vi "Template - Queue1.vi"(7 "Queue Selector":T2=enum."EnQ", 8 "error in (no error)":errorcluster, 10 "Queue1 Data":cluster{"Enum":T1, "Variant":variant}) -> (0 "error out":errorcluster, 2 "Queue Data (out)":cluster{"Enum":T1, "Variant":variant}, 3 "Q1 Ref":T3)   [LabVIEW 2012]
uses:
  TypeDef - Template - Q1 Ref.ctl
  TypeDef - Template - Queue1 Data Enum.ctl
  Navistar Library/Controls/TypeDef - Queue Selector(Standard).ctl
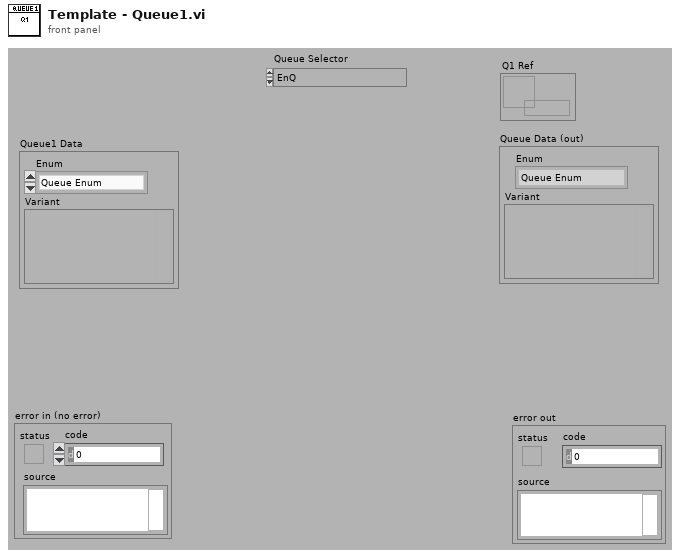
[diagram p1: front panel]
types:
  T1 = typedef "TypeDef - Template - Queue1 Data Enum.ctl" = enum16{"Queue Enum", "Get Time Data", "Check Time", "Stop"}
  T2 = typedef "TypeDef - Queue Selector(Standard).ctl" = enum16{"Create Q", "EnQ", "EnQ at the Opposite", "Flush Q", "Get Q Ref", "Clear Q", "Reset Q"}
  T3 = typedef "TypeDef - Template - Q1 Ref.ctl" = refnum<queue>
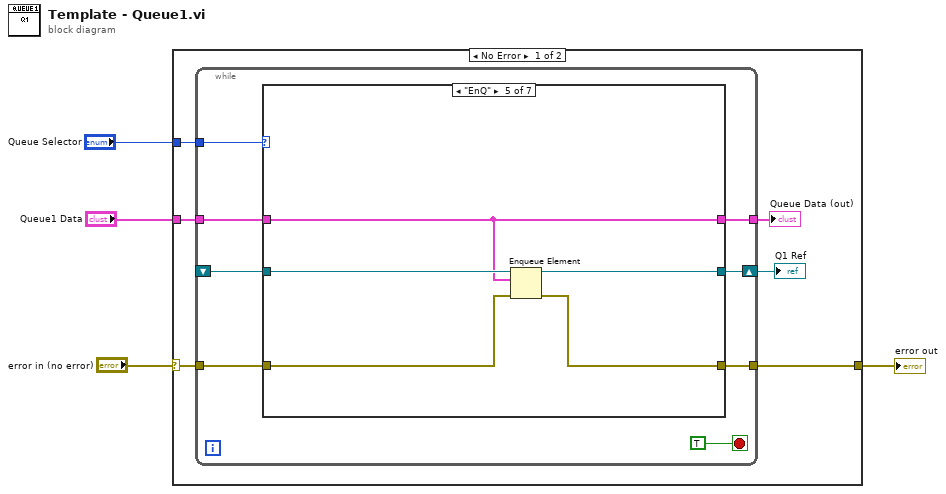
[diagram p0: block diagram]
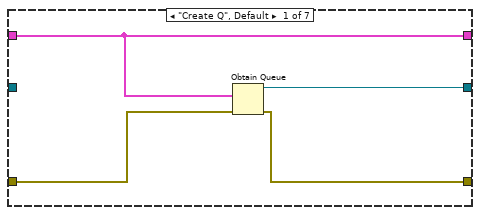
[diagram p2: hidden frame]
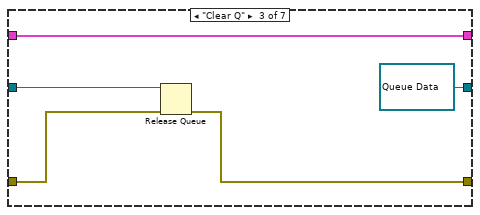
[diagram p4: hidden frame]
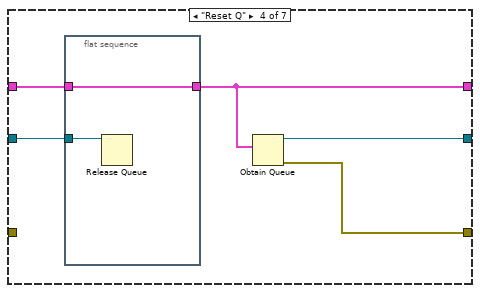
[diagram p5: hidden frame]
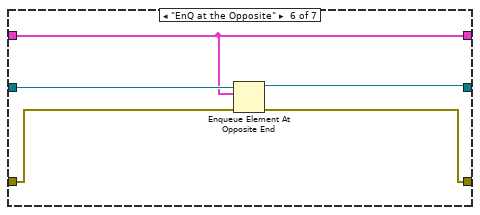
[diagram p6: hidden frame]
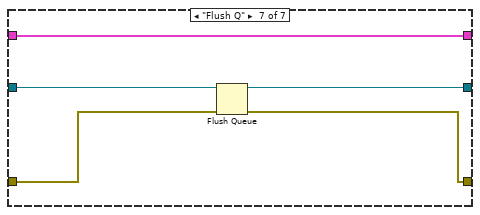
[diagram p7: hidden frame]
diagram:
  n1 = case shown="No Error" "error in (no error)" {
    selector: "error in (no error)" -> [w10 w53]
    tunnel: [w9 w53] -> w3
    tunnel: "Queue Selector" -> [w8 _]
    tunnel: "Queue1 Data" -> [w7 _]
    frame No Error {
      n2 = while {
        shift-right: [w18] -> w6
        shift-left: _ -> [w15]
        tunnel: w10 -> [w17]
        tunnel: [w16] -> w9
        tunnel: w7 -> [w12]
        tunnel: w8 -> [w14]
        tunnel: [w11] -> w5
        stop <- TRUE stop-if-true
        n3 = case shown="\"EnQ\"" w14 {
          tunnel: [w21 w25 refnum<queue> refnum ("queue out") w33 w41 w46 w49] -> w18
          tunnel: w17 -> [w22 w24 w27 _ w40 w45 w51]
          tunnel: [w20 w24 w29 w32 w39 w44 w50] -> w16
          tunnel: w15 -> [_ w25 w28 w35 w42 w47 w52]
          tunnel: w12 -> [w19 w23 w26 w34 w38 w43 w48]
          tunnel: [w19 w23 w26 w31 w38 w43 w48] -> w11
          frame "Create Q", Default {
            n4 = Obtain Queue(element data type=w19, error in (no error)=w22) -> (queue out=w21:refnum<queue>, error out=w20:errorcluster)  [unwired: 3 in, 1 out]
          }
          frame "Get Q Ref" {
          }
          frame "Clear Q" {
            n5 = Release Queue(queue=w28, error in (no error)=w27) -> (error out=w29:errorcluster)  [unwired: 1 in, 2 out]
          }
          frame "Reset Q" {
            n6 = flat-sequence {
              tunnel: w35 -> [w37]
              tunnel: w34 -> [w36]
              tunnel: [w36] -> w31
              frame #0 {
                n7 = Release Queue(queue=w37) -> ()  [unwired: 2 in, 3 out]
              }
            }
            n8 = Obtain Queue(element data type=w31) -> (queue out=w33:refnum<queue>, error out=w32:errorcluster)  [unwired: 4 in, 1 out]
          }
          frame "EnQ" {
            n9 = Enqueue Element(queue=w42, element=w38, error in (no error)=w40) -> (queue out=w41:refnum<queue>, error out=w39:errorcluster)  [unwired: 1 in, 1 out]
          }
          frame "EnQ at the Opposite" {
            n10 = Enqueue Element At Opposite End(queue=w47, element=w43, error in (no error)=w45) -> (queue out=w46:refnum<queue>, error out=w44:errorcluster)  [unwired: 1 in, 1 out]
          }
          frame "Flush Q" {
            n11 = Flush Queue(queue=w52, error in (no error)=w51) -> (queue out=w49:refnum<queue>, error out=w50:errorcluster)  [unwired: 1 out]
          }
        }
      }
      "Q1 Ref" <- w6
      "Queue Data (out)" <- w5
    }
    frame Error {
    }
  }
  "error out" <- w3
